vi "HelpOff.vi"(8 "Error In":errorcluster, 11 "reference in":refnum<class "Clippy.lvclass">) -> (0 "Error Out":errorcluster, 3 "reference out":refnum<class "Clippy.lvclass">)   [LabVIEW 2020, in "Clippy.lvclass"]
uses:
  Clippy.lvclass
  AnimationTypes.ctl
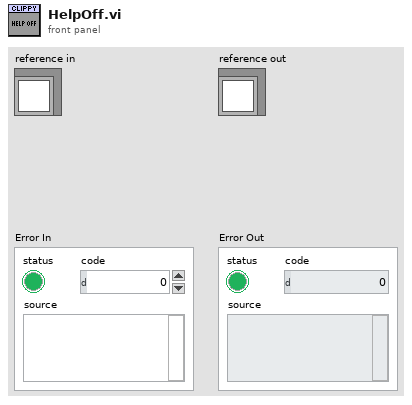
[diagram p1: front panel]
types:
  T1 = typedef "Clippy.lvclass/AnimationTypes.ctl" = enum16{"Congratulate", "LookRight", "SendMail", "Thinking", "Explain", "IdleRopePile", "IdleAtom", "Print", "Hide", "GetAttention", "Save", "GetTechy", "GestureUp", "Idle1_1", "Processing", "Alert", "LookUpRight", "IdleSideToSide", "GoodBye", "LookLeft", "IdleHeadScratch", "LookUpLeft", "CheckingSomething", "Hearing_1", "GetWizardy", "IdleFingerTap", "GestureLeft", "Wave", "GestureRight", "Writing", "IdleSnooze", "LookDownRight", "GetArtsy", "Show", "LookDown", "Searching", "EmptyTrash", "Greeting", "LookUp", "GestureDown", "RestPose", "IdleEyeBrowRaise", "LookDownLeft"}
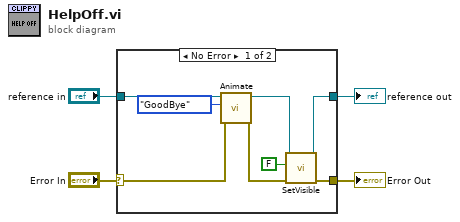
[diagram p0: block diagram]
diagram:
  n1 = case shown="No Error" "Error In" {
    selector: "Error In" -> [w12 w14]
    tunnel: [w8 w14] -> w3
    tunnel: [w5 w13] -> w1
    tunnel: "reference in" -> [w10 w13]
    frame No Error {
      n2 = call-dynamic "Animate.vi"("Error In"=w12, "Animation"=AnimationTypes."GoodBye", "reference in"=w10) -> ("Error Out"=w7:errorcluster, "reference out"=w6:refnum<class "Clippy.lvclass">)  [unwired: 7 in]
      n3 = call "SetVisible.vi"("Error In"=w7, "Visible"=FALSE, "reference in"=w6) -> ("Error Out"=w8:errorcluster, "reference out"=w5:refnum<class "Clippy.lvclass">)  [unwired: 7 in]
    }
    frame Error {
    }
  }
  "Error Out" <- w3
  "reference out" <- w1
